vi "降采样波形图表显示.vi"() -> ()   [LabVIEW 2012]
panel:
  in  "n":i32=2
  in  "stop":bool
  out "随机数波形图表":dbl(graph)
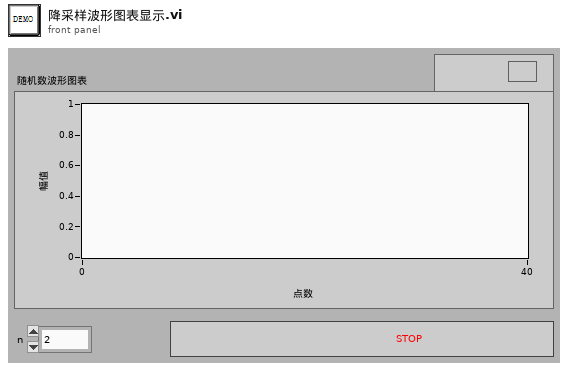
[diagram p1: front panel]
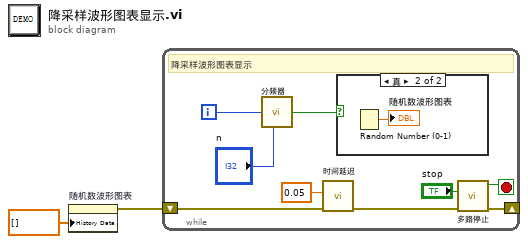
[diagram p0: block diagram]
diagram:
  n1 = property on="随机数波形图表" class="WFChart (严格)"("History Data"=dbl[] [] ("历史数据")) -> (error out=w2:errorcluster)  [unwired: 2 in, 1 out]
  n2 = while {
    shift-right: [w5] -> _
    shift-left: w2 -> [w9]
    i -> [w8]
    stop <- w3 stop-if-true
    # "降采样波形图表显示"
    n3 = call-poly "分频器.vi"("In"=w8, "n"="n") -> ("Out"=w7:bool)  [unwired: 5 in]
    n4 = call "时间延迟"("error in (no error)"=w9, "Delay Time (s)"=0.05) -> ("error out"=w11:errorcluster)  [unwired: 9 in]
    n5 = case shown="真" w7 {
      frame False {
      }
      frame True {
        n6 = Random Number (0-1)() -> (number: 0 to 1=→"随机数波形图表":dbl)
      }
    }
    n7 = call "多路停止.vi"("error in (no error)"=w11, "停止1"="stop") -> ("error in (no error)"=w5:errorcluster, "为真停止"=w3:bool)  [unwired: 6 in, 1 out]
  }
